vi "Cyclic Message Schedule Table Initialize.vi"(8 "error in":errorcluster) -> (0 "error out":errorcluster {"code" min=0 max=0}, 3 "reference out":T1)   [LabVIEW 2013, in "J1939.lvlib"]
uses:
  J1939.lvlib
  Cyclic Frame Scheduler Lut Reference.ctl
  Cyclic Frame Scheduler LUT Command.ctl
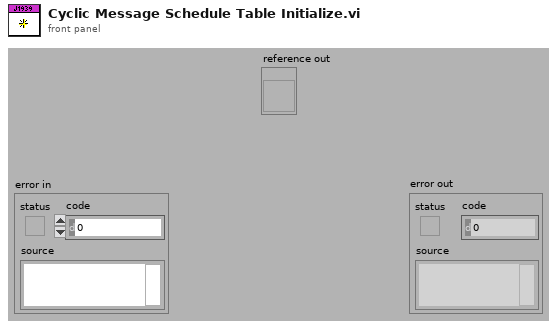
[diagram p1: front panel]
types:
  T1 = typedef "J1939.lvlib/cyclic frame scheduler lut reference.ctl" = refnum<vi>
  T2 = typedef "J1939.lvlib/cyclic frame scheduler lut command.ctl" = enum16{"Initialize", "set", "remove", "calculate times"}
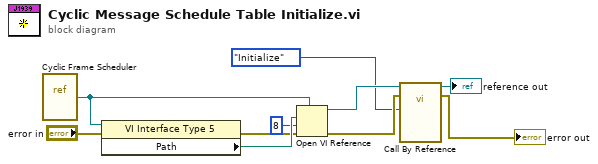
[diagram p0: block diagram]
diagram:
  n1 = vi-ref "Cyclic Frame Scheduler.vi"() -> (w10:refnum<vi>)
  n2 = property class="VI Interface Type 5"(reference=w10, error in="error in") -> (error out=w7:errorcluster, "Path"=w9:path)  [unwired: 1 out]
  n3 = Open VI Reference(type specifier VI Refnum (for type only)=w10, vi path=w9, options=8, error in (no error)=w7) -> (vi reference=w6:refnum<vi>, error out=w3:errorcluster)  [unwired: 2 in]
  n4 = call-by-ref "?"(reference=w6, error in=w3, "command"=cyclic_frame_scheduler_lut_command."Initialize") -> (reference out=→"reference out":refnum<vi>, error out=→"error out":errorcluster)  [unwired: 10 in, 1 out]
